vi "Lift Set.vi"() -> ()   [LabVIEW 2017]
uses:
  Lift Control Type.ctl
  Lift Enum States.ctl
  <vilib>/Rock Robotics/WPI/DriverStation/WPI_DriverStationRobotMode2.ctl
  Lift Globals.vi
  Robot Global Data.vi
panel:
  out "error out 2":errorcluster
  out "error out":errorcluster
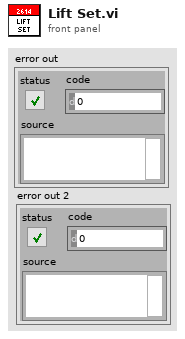
[diagram p1: front panel]
types:
  T1 = typedef "Lift Enum States.ctl" = enum16{"Climb", "Load", "Portal", "Switch", "Scale High", "Scale Mid", "Scale Low", "Exchange", "Stow", "Current Position"}
  T2 = typedef "WPI_DriverStationRobotMode2.ctl" = enum16{"Autonomous Disabled", "Autonomous Enabled", "Teleop Disabled", "Teleop Enabled", "Disconnected", "Finish", "Test Disabled", "Test Enabled", "Emergency Stopped"}
  T3 = typedef "Lift Control Type.ctl" = enum16{"No Op", "Position", "Climb Actuation", "Manual Up", "Manual Down", "PositionAuto", "Position_kP", "Position_Delay"}
  T4 = typedef "Lift Notifier.ctl" = cluster{"Lift Control Type":T3, "Step":i32, "Set Position":T1, "Climb":bool, "Switch":bool, "Scale Low":bool, "Scale Mid":bool, "Scale High":bool, "Stow":bool, "Load":bool, "Climb Actuation":bool, "Manual Up":bool, "Manual Down":bool, "Parameter 1":dbl, "Parameter 2":dbl, "Parameter 3":dbl, "Lift Notifier":refnum<notifier>, "Exchange":bool, "Brake":bool, "Portal":bool}
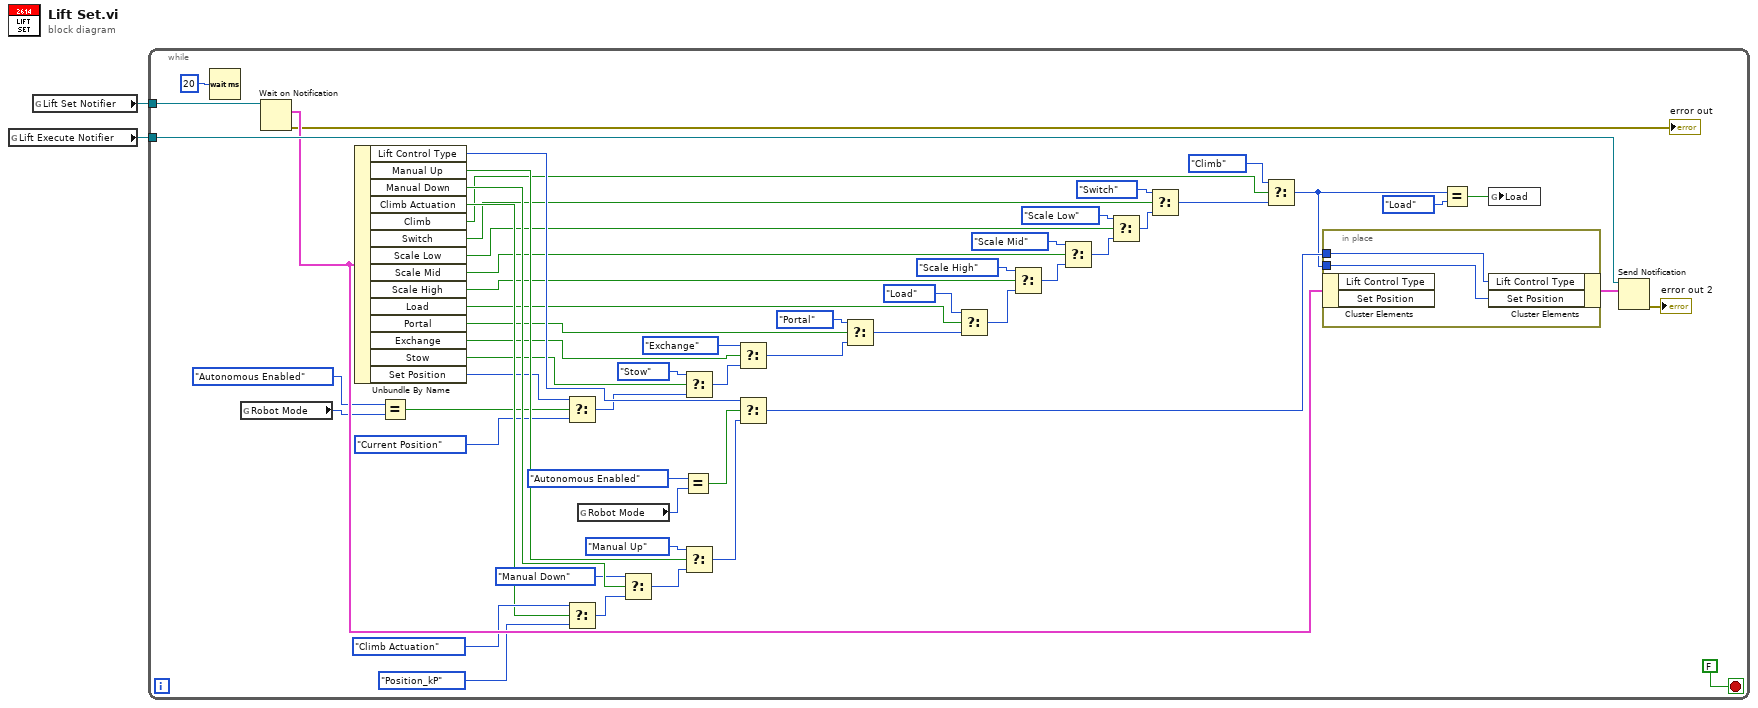
[diagram p0: block diagram]
diagram:
  n1 = global read "Lift Globals.vi" "Lift Execute Notifier"() -> (w2:refnum<notifier>)
  n2 = global read "Lift Globals.vi" "Lift Set Notifier"() -> (w1:refnum<notifier>)
  n3 = while {
    tunnel: w1 -> [w57]
    tunnel: w2 -> [w56]
    stop <- FALSE stop-if-true
    n4 = Wait (ms)(milliseconds to wait=u32 20) -> ()  [unwired: 1 out]
    n5 = global read "Robot Global Data.vi" "Robot Mode"() -> (w22:T2)
    n6 = Wait on Notification(notifier=w57) -> (notification=w55:T4, error out=→"error out":errorcluster)  [unwired: 3 in, 2 out]
    n7 = Unbundle By Name(w55) -> ("Lift Control Type"=w53:T3, "Manual Up"=w47:bool, "Manual Down"=w46:bool, "Climb Actuation"=w42:bool, "Climb"=w17:bool, "Switch"=w16:bool, "Scale Low"=w15:bool, "Scale Mid"=w14:bool, "Scale High"=w13:bool, "Load"=w12:bool, "Portal"=w3:bool, "Exchange"=w11:bool, "Stow"=w10:bool, "Set Position"=w20:T1)
    n8 = Equal?(x=WPI_DriverStationRobotMode2."Autonomous Enabled", y=w22) -> (x = y?=w21:bool)
    n9 = Select(t=w20, s=w21, f=Lift_Enum_States."Current Position" ("Set Position")) -> (s? t:f=w25:T1)
    n10 = Select(t=Lift_Control_Type."Climb Actuation" ("Lift Control Type"), s=w42, f=Lift_Control_Type."Position_kP" ("Lift Control Type")) -> (s? t:f=w41:T3)
    n11 = global read "Robot Global Data.vi" "Robot Mode"() -> (w51:T2)
    n12 = Select(t=Lift_Control_Type."Manual Down" ("Lift Control Type"), s=w46, f=w41) -> (s? t:f=w48:T3)
    n13 = Equal?(x=WPI_DriverStationRobotMode2."Autonomous Enabled", y=w51) -> (x = y?=w52:bool)
    n14 = Select(t=Lift_Enum_States."Stow", s=w10, f=w25) -> (s? t:f=w34:T1)
    n15 = Select(t=Lift_Control_Type."Manual Up" ("Lift Control Type"), s=w47, f=w48) -> (s? t:f=w49:T3)
    n16 = Select(t=Lift_Enum_States."Exchange" ("Set Position"), s=w11, f=w34) -> (s? t:f=w4:T1)
    n17 = Select(t=w53, s=w52, f=w49) -> (s? t:f=w54:T3)
    n18 = Select(t=Lift_Enum_States."Portal" ("Set Position"), s=w3, f=w4) -> (s? t:f=w5:T1)
    n19 = Select(t=Lift_Enum_States."Load", s=w12, f=w5) -> (s? t:f=w36:T1)
    n20 = Select(t=Lift_Enum_States."Scale High", s=w13, f=w36) -> (s? t:f=w37:T1)
    n21 = Select(t=Lift_Enum_States."Scale Mid", s=w14, f=w37) -> (s? t:f=w38:T1)
    n22 = Select(t=Lift_Enum_States."Scale Low", s=w15, f=w38) -> (s? t:f=w39:T1)
    n23 = Select(t=Lift_Enum_States."Switch", s=w16, f=w39) -> (s? t:f=w40:T1)
    n24 = Select(t=Lift_Enum_States."Climb", s=w17, f=w40) -> (s? t:f=w9:T1)
    n25 = in-place {
      in-place-border: w54 -> [w62]
      in-place-border: w9 -> [w61]
      n26 = in-place-cluster #1(w55) -> ()  [unwired: 2 out]
      n27 = in-place-cluster #1("Lift Control Type"=w62, "Set Position"=w61) -> (w58:T4)
    }
    n28 = Equal?(x=w9, y=Lift_Enum_States."Load") -> (x = y?=w7:bool)
    n29 = global write "Lift Globals.vi" "Load"(w7) -> ()
    n30 = Send Notification(notification=w58, notifier=w56) -> (error out=→"error out 2":errorcluster)  [unwired: 1 in, 1 out]
  }
